vi "DCIMG_to_H5_converter.vi"() -> ()   [LabVIEW 2021]
uses:
  <vilib>/addons/h5labview2/file/H5Fmode.ctl
  <vilib>/addons/h5labview2/base/lib_path.vi
  <vilib>/addons/h5labview2/base/H5Equery.vi
  <vilib>/addons/h5labview2/dataset/H5Dwrite.llb/H5Dwrite.xnode
  <vilib>/addons/h5labview2/file/H5F.lvlib
panel:
  in  "Delete DCIMG?":bool
  in  "Move dcimg?":bool=TRUE
  out "Current file number":i32
  in  "Convert to H5?":bool=TRUE
  out "Min / image":dbl
  out "Full run time (min)":u32
  out "Loop #":i32
  out "Saved H5 path":path
  out "Frame":i32
  out "Opened DCIMG path":path
  in  "End experiment":bool
  out "File number":i32
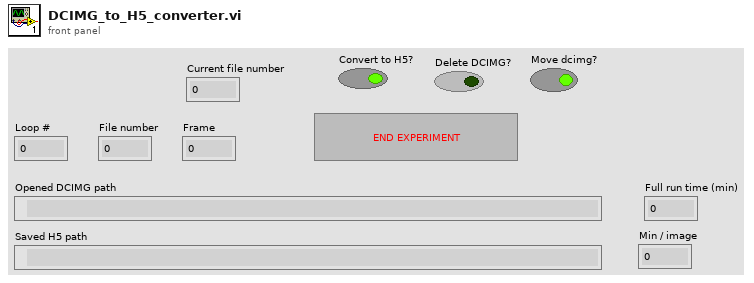
[diagram p1: front panel]
types:
  T1 = typedef "H5F.lvlib/H5Fmode.ctl" = enum16{"read-only", "read-write", "overwrite", "create new", "open or create"}
  T2 = typedef "hid_t.ctl" = i64
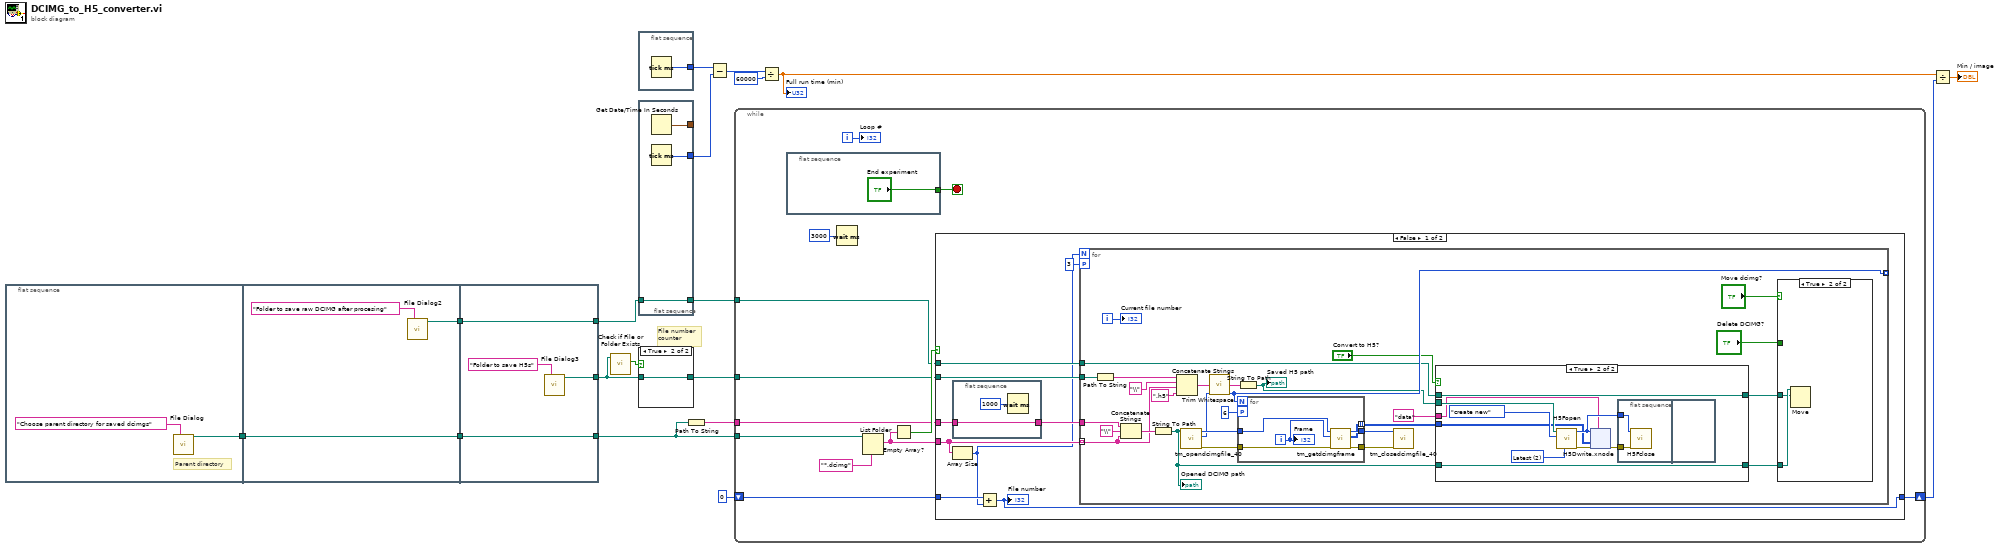
[diagram p0: block diagram]
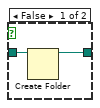
[diagram p2: hidden frame]
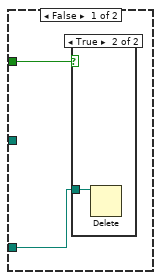
[diagram p3: hidden frame]
diagram:
  # "File number\ncounter"
  n1 = flat-sequence {
    tunnel: [w19] -> w5
    tunnel: w5 -> [w23]
    tunnel: [w23] -> w3
    tunnel: [w21] -> w2
    tunnel: [w26] -> w4
    tunnel: [w27] -> w6
    tunnel: w3 -> [w27]
    tunnel: w2 -> [w26]
    tunnel: [w25] -> w1
    frame #0 {
      # "Parent directory"
      n2 = call "File Dialog"("prompt"="Choose parent directory for saved dcimgs") -> ("selected path"=w19:path)  [unwired: 11 in, 3 out]
    }
    frame #1 {
      n3 = call "File Dialog2"("prompt"="Folder to save raw DCIMG after procesing") -> ("selected path"=w21:path)  [unwired: 11 in, 3 out]
    }
    frame #2 {
      n4 = call "File Dialog3"("prompt"="Folder to save H5s") -> ("selected path"=w25:path)  [unwired: 11 in, 3 out]
    }
  }
  n5 = call <vilib>:"Check if File or Folder Exists.vi"("path"=w1) -> ("file or folder exists?"=w15:bool)  [unwired: 8 in, 2 out]
  n6 = flat-sequence {
    tunnel: [w28] -> w13
    frame #0 {
      n7 = Tick Count (ms)() -> (millisecond timer value=w28:u32)
    }
  }
  n8 = flat-sequence {
    tunnel: w4 -> [w31]
    tunnel: [w31] -> w14
    tunnel: [w30] -> w10
    tunnel: [w29] -> _
    frame #0 {
      n9 = Get Date/Time In Seconds() -> (seconds since 1Jan1904=w29:timestamp)
      n10 = Tick Count (ms)() -> (millisecond timer value=w30:u32)
    }
  }
  n11 = case shown="True" w15 {
    tunnel: w1 -> [w33 w34]
    tunnel: [w32 w34] -> w16
    frame False {
      n12 = Create Folder(path (use dialog)=w33) -> (created path=w32:path)  [unwired: 2 in, 2 out]
    }
    frame True {
    }
  }
  n13 = Path To String(path=w6) -> (string=w17:string)
  n14 = Subtract(x=w13, y=w10) -> (x-y=w11:u32)
  n15 = while {
    tunnel: w14 -> [w39]
    tunnel: w16 -> [w40]
    tunnel: w6 -> [w45]
    tunnel: w17 -> [w41]
    shift-right: [w36] -> w8
    shift-left: 0 -> [w35]
    i -> [w37]
    stop <- w38 stop-if-true
    n16 = flat-sequence {
      tunnel: ["End experiment"] -> w38
      frame #0 {
      }
    }
    n17 = Wait (ms)(milliseconds to wait=u32 3000) -> ()  [unwired: 1 out]
    n18 = List Folder(path=w45, pattern="*.dcimg") -> (filenames=w43:string[])  [unwired: 2 in, 3 out]
    n19 = Empty Array?(array=w43) -> (empty?=w42:bool)
    n20 = case shown="False" w42 {
      tunnel: w43 -> [w52 _]
      tunnel: w41 -> [w53 _]
      tunnel: w40 -> [w56 _]
      tunnel: w39 -> [w55 _]
      tunnel: w35 -> [w51 w130]
      tunnel: [w49 w130] -> w36
      frame False {
        n21 = flat-sequence {
          tunnel: [w57] -> w54
          tunnel: w53 -> [w57]
          frame #0 {
            n22 = Wait (ms)(milliseconds to wait=u32 1000) -> ()  [unwired: 1 out]
          }
        }
        n23 = Array Size(array=w52) -> (size(s)=w50:i32)
        n24 = Add(x=w51, y=w50) -> (x+y=w49:i32)
        "File number" <- w49
        n25 = for {
          N: w50 -> [_]
          tunnel: [w80] -> _ mode=indexing
          tunnel: w52 -> [w70] mode=indexing
          tunnel: w54 -> [w78]
          tunnel: w56 -> [w75]
          tunnel: w55 -> [w66]
          workers-P: 3 -> [_]
          i -> [w65]
          n26 = Path To String(path=w75) -> (string=w73:string)
          n27 = Concatenate Strings(w78, "\\" ("string"), w70) -> (w77:string)
          n28 = String To Path(string=w77) -> (path=w67:path)
          "Opened DCIMG path" <- w67
          n29 = Concatenate Strings(w73, "\\" ("string"), w70, ".h5") -> (w76:string)
          n30 = call <userlib>:"tm_opendcimgfile_40.vi"("Path"=w67) -> ("error out"=w83:errorcluster, "Total Frames"=w80:i32, "File Handle"=w85:u32)  [unwired: 8 in]
          n31 = call <vilib>:"Trim Whitespace.vi"("string"=w76) -> ("trimmed string"=w81:string)  [unwired: 1 in]
          n32 = for {
            N: w80 -> [_]
            tunnel: w85 -> [w129]
            tunnel: [w128] -> w84
            tunnel: w83 -> [w127]
            tunnel: [w126] -> w82
            workers-P: 6 -> [_]
            tunnel: [w124] -> w68 mode=indexing
            i -> [w125]
            n33 = call <userlib>:"tm_getdcimgframe.vi"("error in (no error)"=w127, "Frame Index"=w125, "File Handle in"=w129) -> ("error out"=w126:errorcluster, "Data"=w124:u16[][], "File Handle out"=w128:u32)  [unwired: 5 in, 1 out]
            "Frame" <- w125
          }
          n34 = String To Path(string=w81) -> (path=w69:path)
          "Saved H5 path" <- w69
          n35 = call <userlib>:"tm_closedcimgfile_40.vi"("error in (no error)"=w82, "File Handle"=w84) -> ()  [unwired: 9 in, 1 out]
          n36 = case shown="True" "Convert to H5?" {
            tunnel: w69 -> [_ w102]
            tunnel: "data" ("dataset name") -> [_ w98]
            tunnel: w68 -> [_ w96]
            tunnel: w67 -> [w91 w94]
            tunnel: w66 -> [w92 w93]
            tunnel: [w91 w94] -> w64
            tunnel: [w92 w93] -> w63
            frame False {
            }
            frame True {
              w99 = u16 2 items=["Earliest", "v1.8", "Latest"] ("compatibility")
              n37 = call <vilib>:"H5Fopen.vi"("compatibility"=w99, "mode (read-only)"=H5Fmode."create new", "path"=w102) -> ("error out"=w97:errorcluster, "ref out"=w101:T2)  [unwired: 7 in]
              n38 = xnode "H5Dwrite.xnode"("dataset name"=w98, "error in (no error)"=w97, "data"=w96, "ref in"=w101) -> ("error out"=w95:errorcluster)  [unwired: 3 in, 2 out]
              n39 = flat-sequence {
                tunnel: w95 -> [w104]
                tunnel: w101 -> [w103]
                frame #0 {
                  n40 = call <vilib>:"H5Fclose.vi"("error in (no error)"=w104, "ref"=w103) -> ()  [unwired: 9 in, 1 out]
                }
                frame #1 {
                }
              }
            }
          }
          n41 = case shown="True" "Move dcimg?" {
            tunnel: w64 -> [w86 w90]
            tunnel: w63 -> [_ w89]
            tunnel: "Delete DCIMG?" -> [w87 _]
            frame False {
              n42 = case shown="True" w87 {
                tunnel: w86 -> [_ w88]
                frame False {
                }
                frame True {
                  n43 = Delete(path (use dialog)=w88) -> ()  [unwired: 4 in, 3 out]
                }
              }
            }
            frame True {
              n44 = Move(source path=w90, 10:w89) -> ()  [unwired: 3 in, 3 out]
            }
          }
          "Current file number" <- w65
        }
      }
      frame True {
      }
    }
    "Loop #" <- w37
  }
  n45 = Divide(x=w11, y=u32 60000) -> (x/y=w9:dbl)
  "Full run time (min)" <- w9
  n46 = Divide(x=w9, y=w8) -> (x/y=→"Min / image":dbl)
